vi "3D Draw.vi"(6 "z vector":dbl[](array[numeric]) format="%.2f", 7 "次数":i32=50, 8 "error in":errorcluster, 9 "y vector":dbl[](array[numeric]) format="%.2f", 10 "x vector":dbl[](array[numeric]) format="%.2f", 11 "3D Ref":refnum<k7>) -> (0 "error out":errorcluster)   [LabVIEW 2020]
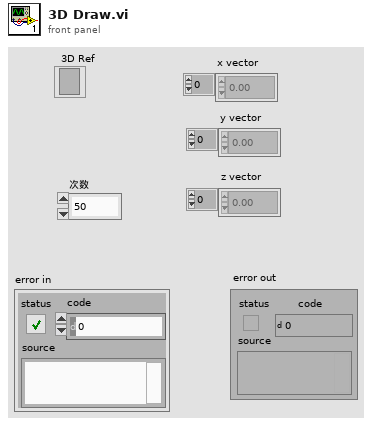
[diagram p1: front panel]
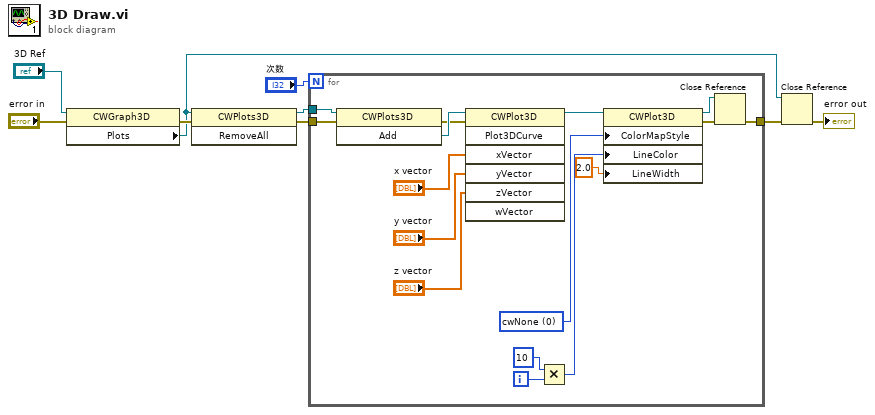
[diagram p0: block diagram]
diagram:
  n1 = property class="CWGraph3D"(reference="3D Ref", error in="error in") -> (error out=w8:errorcluster, "Plots"=w4:refnum<k7>)  [unwired: 1 out]
  n2 = invoke class="CWPlots3D" method="RemoveAll"(reference=w4, error in=w8) -> (reference out=w7:refnum<k7>, error out=w6:errorcluster)  [unwired: 1 in, 1 out]
  n3 = for {
    N: "次数" -> [_]
    tunnel: w7 -> [w25]
    tunnel: w6 -> [w23]
    tunnel: [w13] -> w5
    i -> [w19]
    w20 = 0 items=["cwNone", "cwShaded", "cwColorSpectrum", "cwGrayScale", "cwCustom"] ("ColorMapStyle")
    n4 = invoke class="CWPlots3D" method="Add"(reference=w25, error in=w23) -> (error out=w22:errorcluster, "Add"=w24:refnum<k7>)  [unwired: 1 in, 1 out]
    n5 = invoke class="CWPlot3D" method="Plot3DCurve"(reference=w24, error in=w22, "xVector"="x vector", "yVector"="y vector", "zVector"="z vector") -> (reference out=w21:refnum<k7>)  [unwired: 2 in, 6 out]
    n6 = Multiply(x=10 ("dimension size"), y=w19) -> (x*y=w17:i32)
    n7 = property class="CWPlot3D"(reference=w21, "ColorMapStyle"=w20, "LineColor"=w17, "LineWidth"=2.0) -> (reference out=w14:refnum<k7>, error out=w15:errorcluster)  [unwired: 1 in]
    n8 = Close Reference(reference=w14, error in (no error)=w15) -> (error out=w13:errorcluster)
  }
  n9 = Close Reference(reference=w4, error in (no error)=w5) -> (error out=→"error out":errorcluster)
